vi "Initialize.vi"(8 "error in (no error)":errorcluster, 10 "Top Level Diagram":refnum<vi>, 11 "Structures in":refnum<class "Structures.lvclass">) -> (0 "error out":errorcluster, 3 "Structures out":refnum<class "Structures.lvclass">)   [LabVIEW 2015, in "Structures.lvclass"]
uses:
  Structures.lvclass
  Structures.lvclass/Structures.ctl
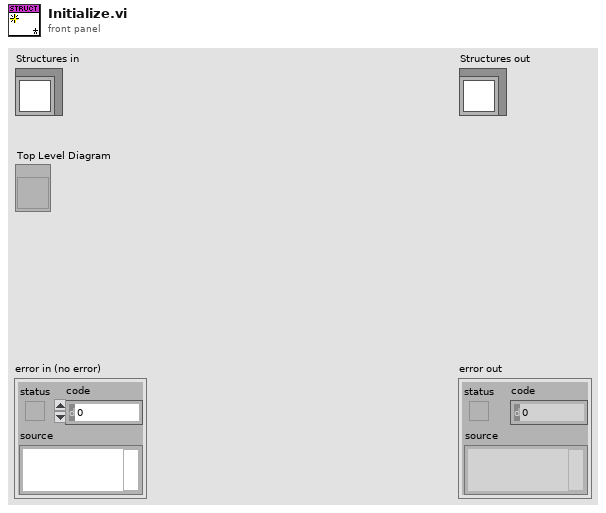
[diagram p1: front panel]
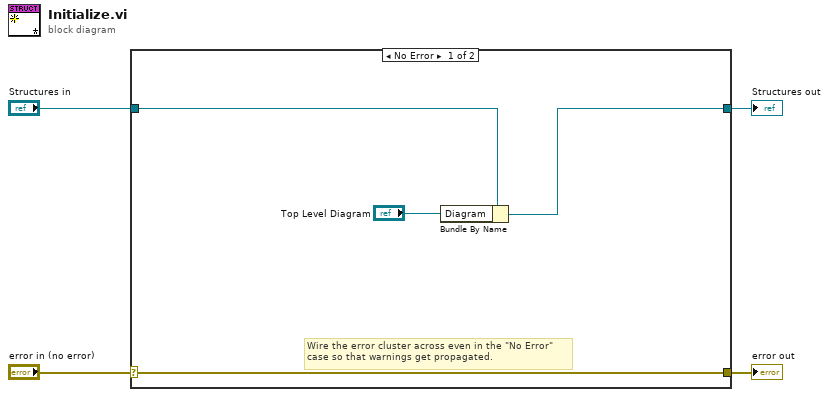
[diagram p0: block diagram]
diagram:
  n1 = case shown="No Error" "error in (no error)" {
    selector: "error in (no error)" -> [w8 w10]
    tunnel: [w8 w10] -> w3
    tunnel: [w6 w9] -> w1
    tunnel: "Structures in" -> [w7 w9]
    frame No Error {
      # "Wire the error cluster across even in the \"No Error\"\ncase so that warnings get propagated."
      n2 = Bundle By Name(cluster=w7, "Diagram"="Top Level Diagram") -> (w6:refnum<class "Structures.lvclass">)
    }
    frame Error {
    }
  }
  "error out" <- w3
  "Structures out" <- w1
